vi "Run main.vi"() -> ()   [LabVIEW 2016]
uses:
  Program Files (x86)/National Instruments/LabVIEW 2016/examples/robotics/EPOS2 CANOpen Driver/Low Level VIs/Typedefs/CAN Refnum.ctl
  Program Files (x86)/National Instruments/LabVIEW 2016/examples/robotics/EPOS2 CANOpen Driver/Low Level VIs/Typedefs/CAN Session Pointer.ctl
  Program Files (x86)/National Instruments/LabVIEW 2016/examples/robotics/EPOS2 CANOpen Driver/Low Level VIs/Typedefs/CAN Communication References.ctl
  Program Files (x86)/National Instruments/LabVIEW 2016/examples/robotics/EPOS2 CANOpen Driver/Low Level VIs/Typedefs/kill process notifier array.ctl
  Program Files (x86)/National Instruments/LabVIEW 2016/examples/robotics/EPOS2 CANOpen Driver/Low Level VIs/Typedefs/Write Queue.ctl
  Program Files (x86)/National Instruments/LabVIEW 2016/examples/robotics/EPOS2 CANOpen Driver/Low Level VIs/Typedefs/FPGA CAN Frame Cluster.ctl
  RT/BMS Voltage status 2.ctl
  Tests/BMS Status.ctl
  RT/Pedals Status.ctl
  RT/Clustered SDO.ctl
  RT/Statusword.ctl
  Tests/Dashboard Control.ctl
  RT/Battery Status.ctl
  Tests/Log File Cluster.ctl
  <vilib>/Platform/TimedLoop/XDataNode/timing_clust.ctl
  <vilib>/Platform/TimedLoop/XDataNode/nitl_modes.ctl
  <vilib>/Platform/TimedLoop/XDataNode/wakeup.ctl
  <vilib>/Platform/TimedLoop/XDataNode/XDataNode.xnode
  <vilib>/Platform/TimedLoop/XDataNode/XDNodeRunTimeDep.lvlib
  <vilib>/NI_Real-Time Target Support.lvlib
panel:
  out "Error Notifier":refnum<notifier>
  out "LED Period":i64
  out "LED Color":i16
  out "Last Pedals Update":u32
  in  "Tab Control":T1(tab)
  in  "Don't irritate me":bool=TRUE
  in  "Simulate BMS LV":bool=TRUE
  in  "Simulate Dashboard":bool=TRUE
  in  "Simulate Pedals":bool=TRUE
  in  "Simulate Motors":bool=TRUE
  in  "Simulation Interval":u32=20
  in  "Simulate BMS":bool=TRUE
  in  "\"Pedals\" Status":T2 {"Acceleration pedal" scale=0.0..100.0 scale format="%#_6f%%"; "Break pedal" scale=0.0..100.0 scale format="%#_6f%%"}
  out "Left Motor Status":T3
  out "Target Torque Left":i16(knob) scale=-1000.0..1000.0
  out "Left Motor Statusword":T4
  out "Right Motor Status":T3
  out "Right Motor Statusword":T4
  out "Target Torque Right":i16(knob) scale=1000.0..-1000.0
  out "BMS Status":T5
  out "Battery Status":T6
  out "BMS Low Voltage Status":T7 {"Temp. 0" scale=0.0..80.0; "Temp. 1" scale=0.0..80.0}
  in  "Ready to drive":bool
  in  "Simulate Pumps":bool
  in  "Pumps power":dbl(slide) scale=0.0..100.0 scale format="%#_g%%"
  in  "Dashboard Control":T8={"Tractive System"=TRUE, "RTD"=TRUE, "AMS error"=TRUE, "IMD error"=TRUE, "Low Voltage"=0.0, "High Voltage"=0.0} {"High Voltage" scale=0.0..10.0; "Low Voltage" scale=0.0..10.0}
  in  "Error Listbox":i32(listbox)
  out "Update motors notifier":i32
  out "Update Motors Notifier":refnum<notifier>
  out "Emergency Turn Off Notifier":refnum<notifier>
  out "Pedals status":i32
  out "Update motors":i32
  out "Pool status":i32
  out "Error Queue":refnum<queue>
  out "Shutdown Notifier":refnum<notifier>
  out "Log File Cluster":T9
  out "CAN Session":T11
  out "CANOpen Session":refnum<k20>
  out "Left motor Clustered SDO":T12
  out "Right motor Clustered SDO":T12
  out "State Ring":u16(ring) items=["Init VI", "Init Event Handlers", "Booting sequence", "Operational", "Emergency shutting down", "Shuting down", "Closing VI"]
  in  "Emergency Shutdown Button":bool
  in  "Shutdown Button":bool
  in  "Stop":bool
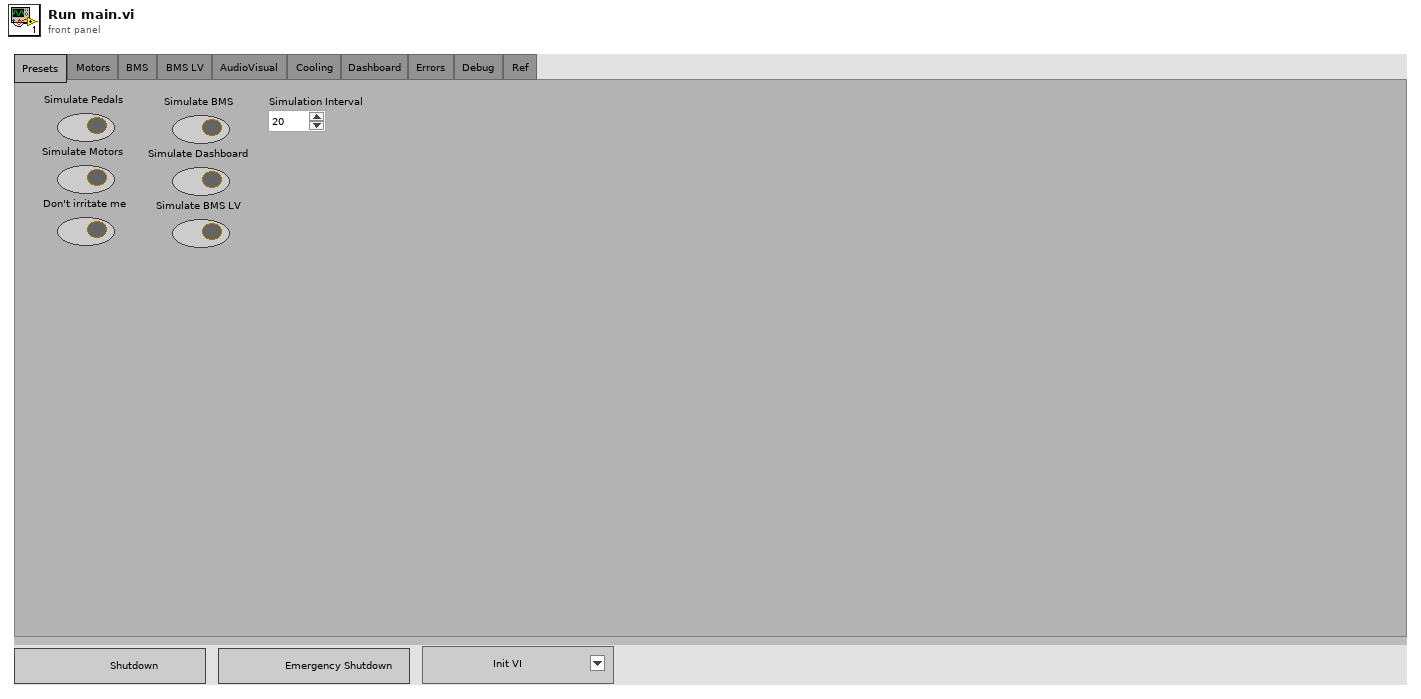
[diagram p1: front panel]
types:
  T1 = enum32{"Presets ", "Motors ", "BMS ", "BMS LV ", "AudioVisual ", "Cooling ", "Dashboard", "Errors ", "Debug ", "Ref "}
  T2 = typedef "Pedals Status.ctl" = cluster{"Acceleration pedal":dbl, "Break pedal":dbl, "Sterring wheel":dbl[unit]}
  T3 = cluster{"Statusword":u16, "Warnings":u16, "Error code":u16, "Error register":u8, "Controller temperature":u8, "Motor temperature":u8, "Troque actual value":i16, "Velocity actual value":i32, "Electric power":u32, "DC current":u32, "Phase A current":u16, "Phase B current":u16, "Electrical Angle":u16}
  T4 = typedef "Statusword.ctl" = cluster{"Ready to switch on":bool, "Switched on":bool, "Operation enabled":bool, "Fault":bool, "Voltage enabled":bool, "Quick stop":bool, "Switch on disabled":bool, "Warning":bool, "Remote":bool, "Target reached":bool, "Internal limit active":bool, "Operation mode specific":bool, "Manufacturer specific":bool}
  T5 = typedef "BMS Status.ctl" = cluster{"INIT":bool, "READY":bool, "WAIT_FOR_ACTIVE":bool, "ACTIVE":bool, "ERROR":bool}
  T6 = typedef "Battery Status.ctl" = cluster{"Hall sensor":i32, "Percent of charge":i16}
  T7 = typedef "BMS Voltage status 2.ctl" = cluster{"Cells Voltage":dbl[], "Temp. 1":u8, "Temp. 0":u8}
  T8 = typedef "Dashboard Control.ctl" = cluster{"Tractive System":bool, "RTD":bool, "AMS error":bool, "IMD error":bool, "Low Voltage":dbl, "High Voltage":dbl}
  T9 = typedef "Log File Cluster.ctl" = cluster{"Log file":refnum<k34>, "semaphore":T10}
  T10 = typedef "Semaphore RefNum" = refnum<k1>
  T11 = typedef "CAN Refnum.ctl" = refnum<k1>
  T12 = typedef "Clustered SDO.ctl" = cluster{"SDO object out":refnum<k20>, "semaphore":T10}
  T13 = typedef "XDNodeRunTimeDep.lvlib/timing_clust.ctl" = cluster{"Expected End [f-1]":u64, "Actual End [f-1]":u64, "Finished Late? [f-1]":bool, "Expected End [i-1]":u64, "Actual End [i-1]":u64, "Finished Late? [i-1]":bool, "Expected Start [i]":u64, "Actual Start [i]":u64, "Expected Start [f]":u64, "Actual Start [f]":u64, "Source Name":string, "Structure Name":string, "Period":i64, "Deadline":i64, "Offset":i64, "Start":i64, "Priority":i32, "Timeout":i32, "Mode":T14, "Wakeup Reason":T15, "Error":errorcluster, "Source Type":string, "Secondary Source Type":string, "Global End Time":u64, "Global Start Time":u64, "Frame Duration":u64, "Iteration Duration":u64, "Assigned CPU":i32, "I/O Scan Engine Mode":u32}
  T14 = typedef "XDNodeRunTimeDep.lvlib/nitl_modes.ctl" = enum32{"No Change", "Process missed periods, maintain original phase", "Discard missed periods, maintain original phase", "Process missed periods, ignore original phase", "Discard missed periods, ignore original phase"}
  T15 = typedef "XDNodeRunTimeDep.lvlib/wakeup.ctl" = enum32{"Normal", "Aborted", "Asynchronous wakeup", "Timing source error", "Timed loop error", "Timeout"}
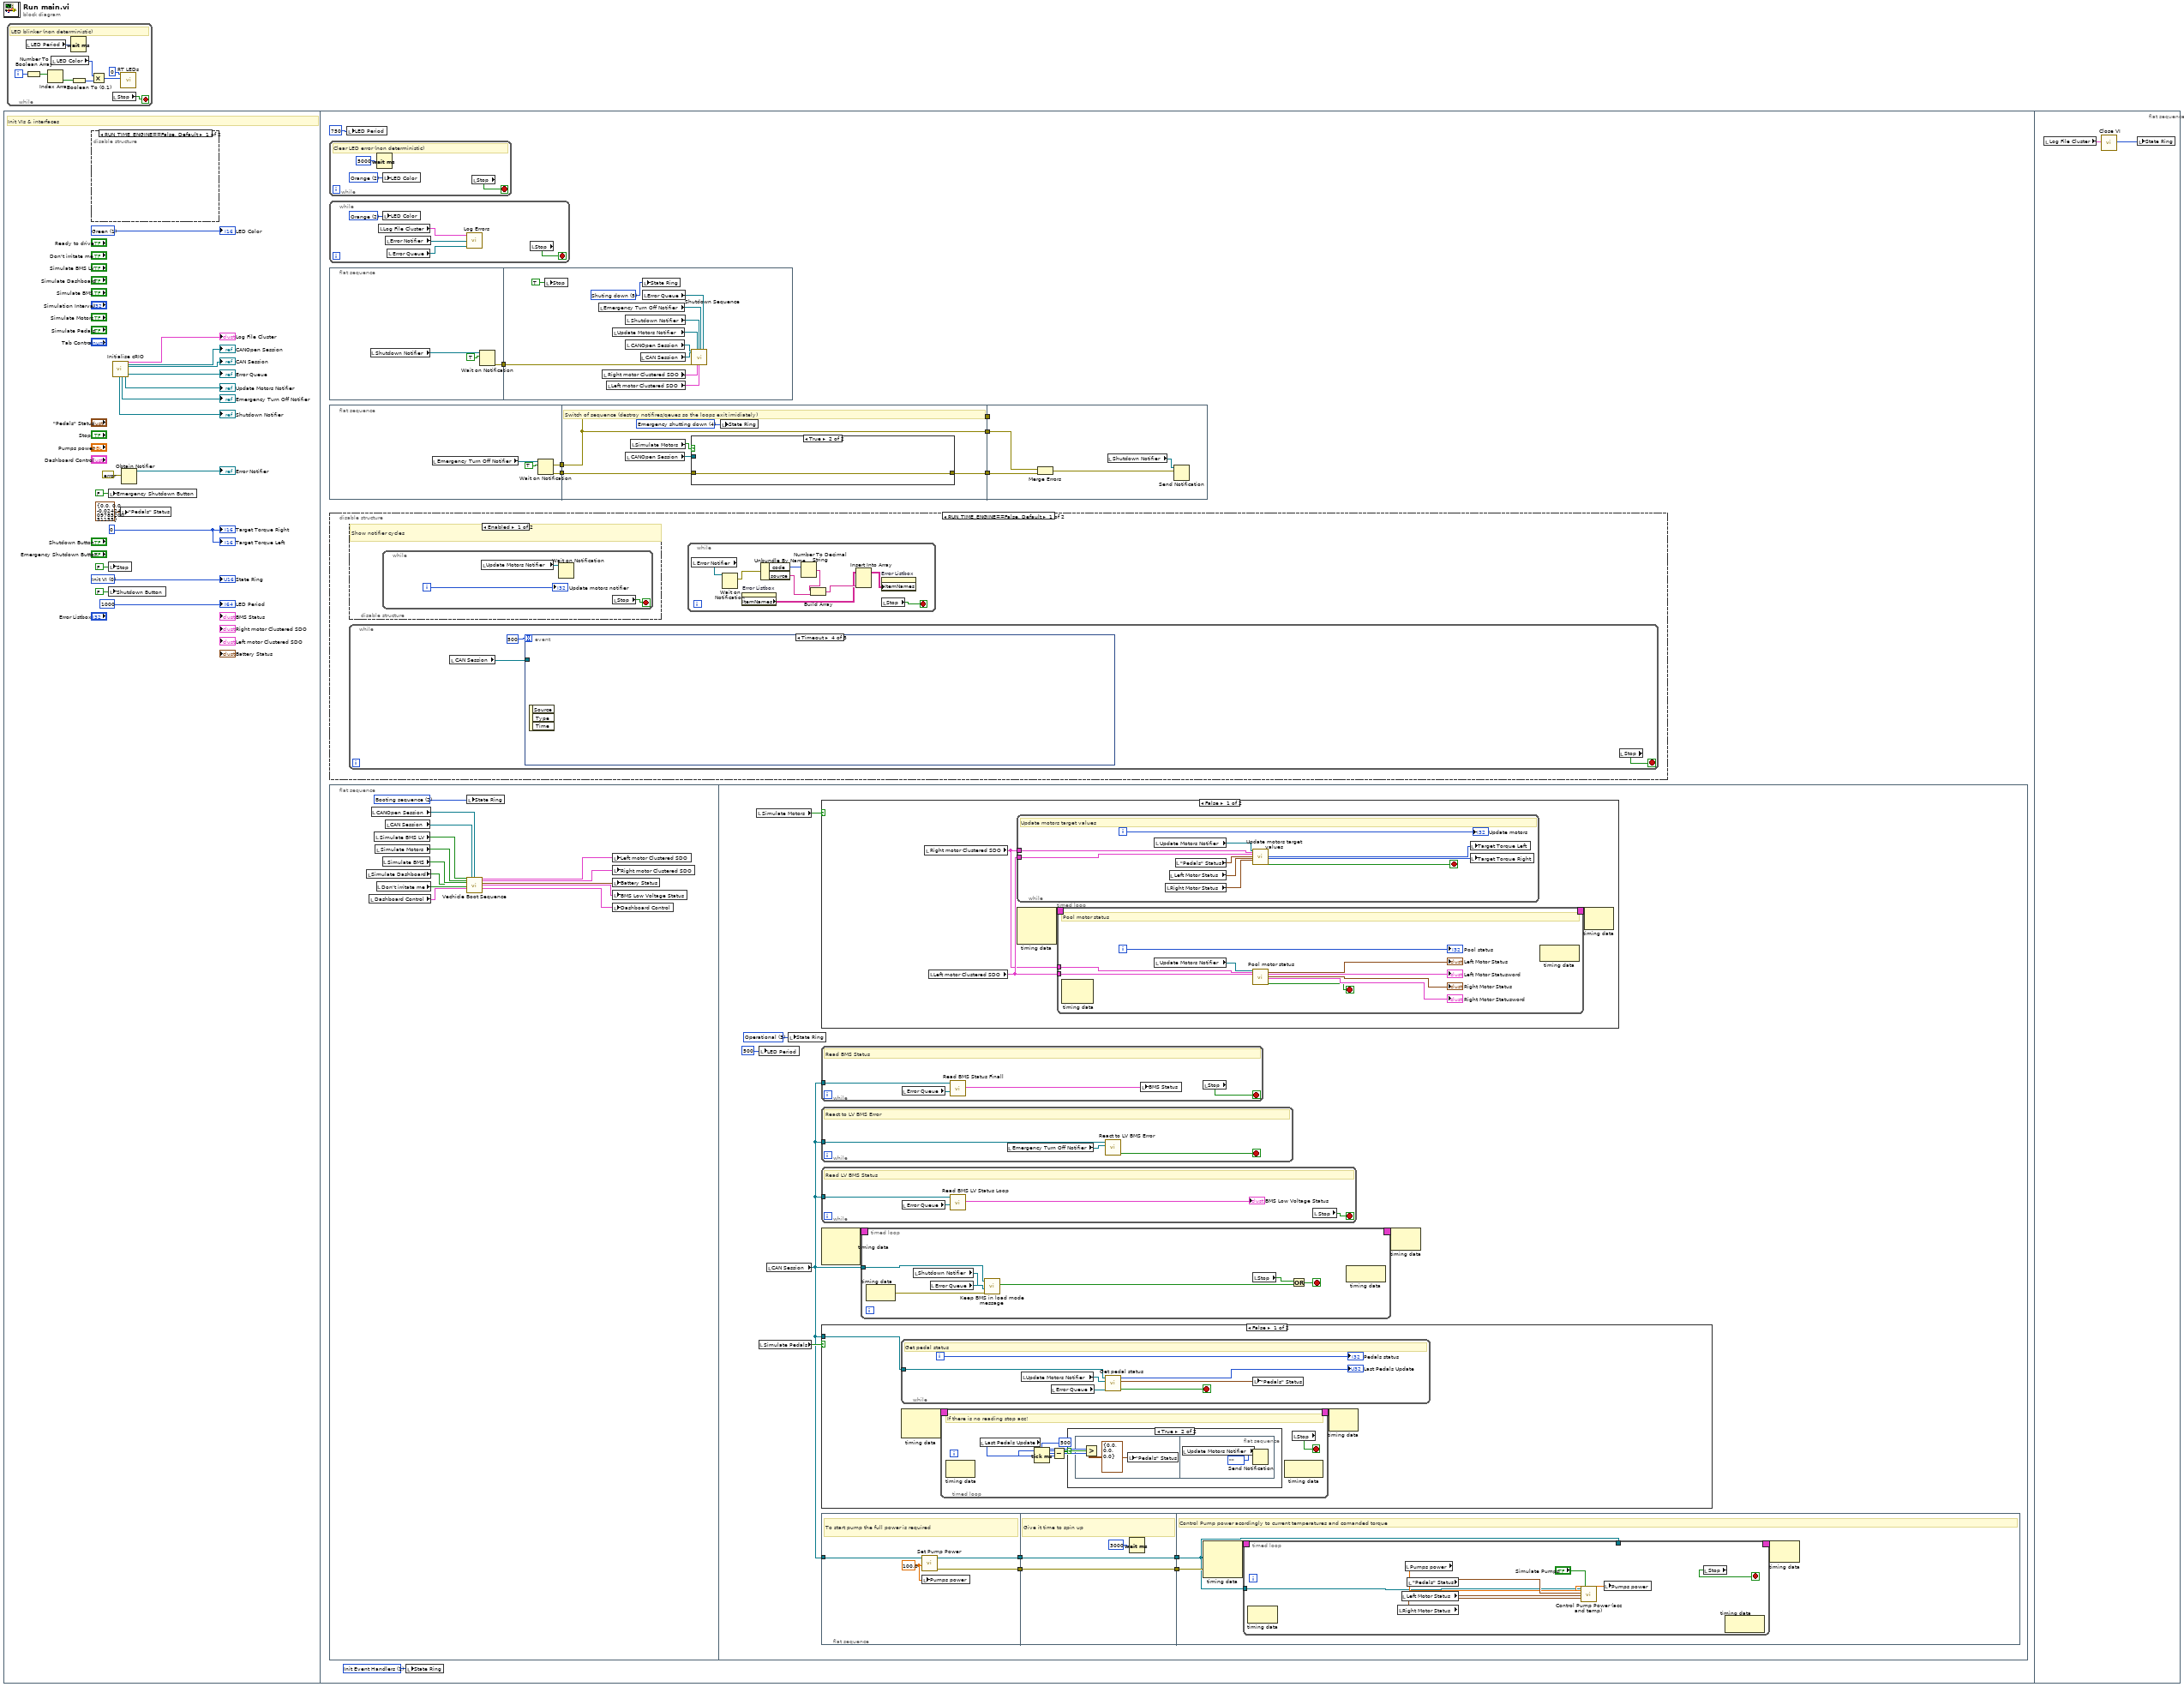
[diagram p0: block diagram]
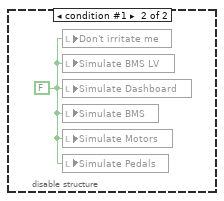
[diagram p2: hidden frame]
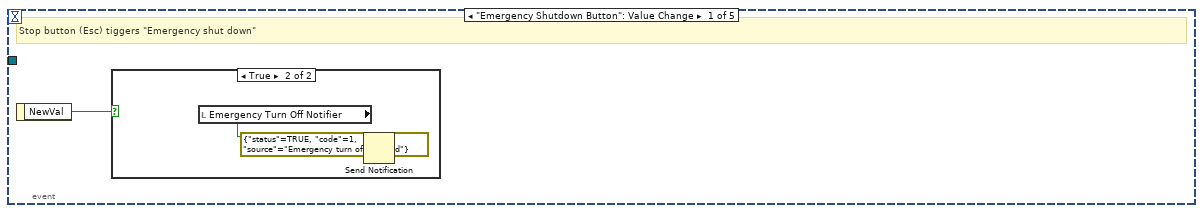
[diagram p4: hidden frame]
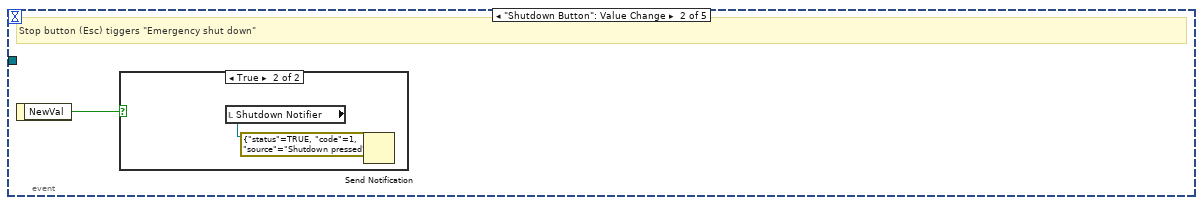
[diagram p6: hidden frame]
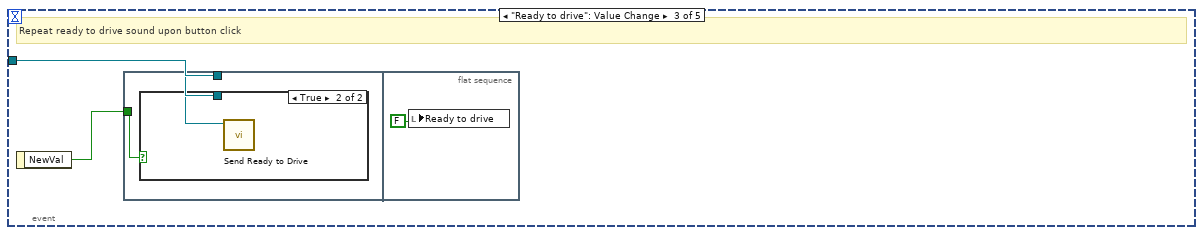
[diagram p8: hidden frame]
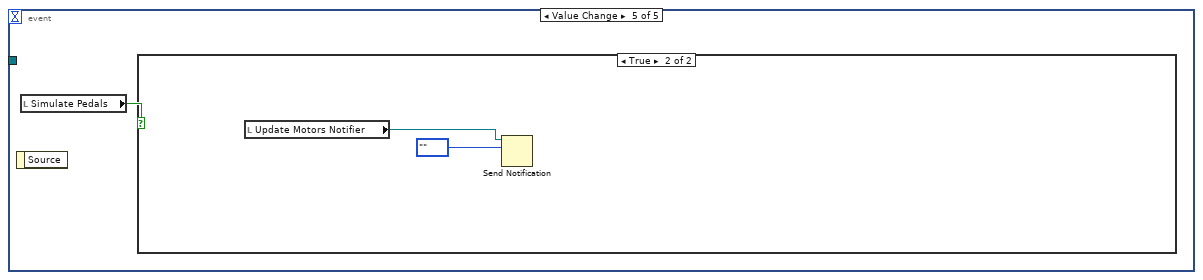
[diagram p10: hidden frame]
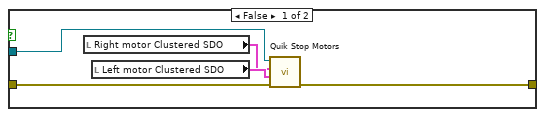
[diagram p13: hidden frame]
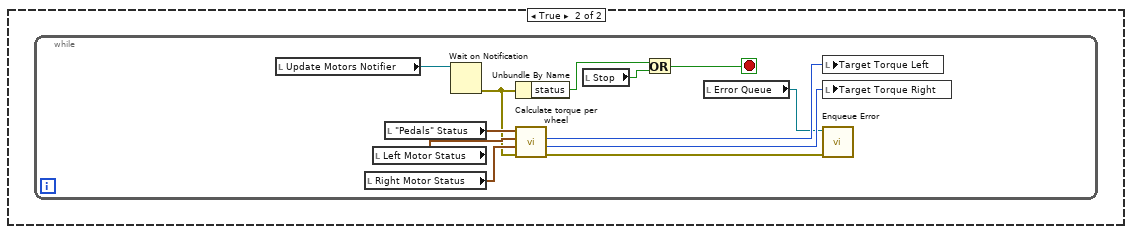
[diagram p16: hidden frame]
diagram:
  n1 = flat-sequence {
    frame #0 {
      w7 = u16 0 items=["Init VI", "Init Event Handlers", "Booting sequence", "Operational", "Emergency shutting down", "Shuting down", "Closing VI"] ("State Ring")
      w9 = u16 1 items=["Green"=1, "Orange"=2]
      w11 = i16 0 ("Target Torque")
      # "Init VIs & interfaces"
      n2 = disable-structure shown="RUN_TIME_ENGINE==False, Default" {
        frame condition #0 (active) {
        }
        frame condition #1 {
          w18 = FALSE ("Don't irritate me")
          n3 = local write "Don't irritate me"(w18) -> ()
          n4 = local write "Simulate BMS LV"(w18) -> ()
          n5 = local write "Simulate Dashboard"(w18) -> ()
          n6 = local write "Simulate BMS"(w18) -> ()
          n7 = local write "Simulate Motors"(w18) -> ()
          n8 = local write "Simulate Pedals"(w18) -> ()
        }
      }
      n9 = local write "Emergency Shutdown Button"(FALSE ("Emergency Shutdown Button")) -> ()
      n10 = local write "Stop"(FALSE ("Stop")) -> ()
      n11 = local write "Shutdown Button"(FALSE ("Shutdown Button")) -> ()
      n12 = call "Initialise cRIO.vi"() -> ("Shutdown Notifier"=→"Shutdown Notifier":refnum<notifier>, "Emergency Turn Off Notifier"=→"Emergency Turn Off Notifier":refnum<notifier>, "Update Motors Notifier"=→"Update Motors Notifier":refnum<notifier>, "Log File Cluster"=→"Log File Cluster":T9, "CANOpen Session"=→"CANOpen Session":refnum<k20>, "CAN Session"=→"CAN Session":T11, "Error Queue"=→"Error Queue":refnum<queue>)  [unwired: 20 in, 1 out]
      n13 = local write "\"Pedals\" Status"(T2 {"Acceleration pedal"=0.0, "Break pedal"=0.0, "Sterring wheel"=-0.024240978520051155} ("\"Pedals\" Status")) -> ()
      n14 = Obtain Notifier(notification data type=errorcluster {"status"=FALSE, "code"=0, "source"=""} ("error constant")) -> (notifier out=→"Error Notifier":refnum<notifier>)  [unwired: 3 in, 2 out]
      "Target Torque Left" <- w11
      "Target Torque Right" <- w11
      "LED Color" <- w9
      "LED Period" <- i64 1000 ("LED Period")
      "State Ring" <- w7
    }
    frame #1 {
      w19 = u16 1 items=["Init VI", "Init Event Handlers", "Booting sequence", "Operational", "Emergency shutting down", "Shuting down", "Closing VI"] ("State Ring")
      n15 = while {
        stop <- w28 stop-if-true
        w29 = u16 2 items=["Green"=1, "Orange"=2]
        # "Clear LED error (non deterministic)"
        n16 = Wait (ms)(milliseconds to wait=u32 5000) -> ()  [unwired: 1 out]
        n17 = local write "LED Color"(w29) -> ()
        n18 = local read "Stop"() -> (w28:bool)
      }
      n19 = while {
        stop <- w34 stop-if-true
        w32 = u16 2 items=["Green"=1, "Orange"=2]
        n20 = local read "Log File Cluster"() -> (w31:T9)
        n21 = local write "LED Color"(w32) -> ()
        n22 = local read "Error Notifier"() -> (w30:refnum<notifier>)
        n23 = local read "Error Queue"() -> (w33:refnum<queue>)
        n24 = call "Log Errors.vi"("Error Queue"=w33, "Error Notifier"=w30, "Log File Cluster"=w31) -> ()  [unwired: 1 in]
        n25 = local read "Stop"() -> (w34:bool)
      }
      n26 = flat-sequence {
        tunnel: [w65] -> w23
        tunnel: w23 -> [w72]
        frame #0 {
          n27 = local read "Shutdown Notifier"() -> (w66:refnum<notifier>)
          n28 = Wait on Notification(notifier=w66, ignore previous (F)=TRUE) -> (error out=w65:errorcluster)  [unwired: 2 in, 3 out]
        }
        frame #1 {
          w68 = u16 5 items=["Init VI", "Init Event Handlers", "Booting sequence", "Operational", "Emergency shutting down", "Shuting down", "Closing VI"] ("State Ring")
          n29 = local write "Stop"(TRUE ("Stop")) -> ()
          n30 = local read "Emergency Turn Off Notifier"() -> (w69:refnum<notifier>)
          n31 = local read "Right motor Clustered SDO"() -> (w73:T12)
          n32 = local read "Left motor Clustered SDO"() -> (w74:T12)
          n33 = local read "Update Motors Notifier"() -> (w76:refnum<notifier>)
          n34 = local read "Shutdown Notifier"() -> (w75:refnum<notifier>)
          n35 = local read "CANOpen Session"() -> (w78:refnum<k20>)
          n36 = local read "CAN Session"() -> (w77:T11)
          n37 = local write "State Ring"(w68) -> ()
          n38 = local read "Error Queue"() -> (w71:refnum<queue>)
          n39 = call "Shutdown Sequence.vi"("CANOpen Session"=w78, "CAN Session"=w77, "error in (no error)"=w72, "Update Motors Notifier"=w76, "Right motor Clustered SDO"=w73, "Shutdown Notifier"=w75, "Left motor Clustered SDO"=w74, "Emergency Turn Off Notifier"=w69, "Error Queue"=w71) -> ()  [unwired: 18 in, 1 out]
        }
      }
      n40 = flat-sequence {
        tunnel: [w81] -> w26
        tunnel: [w80] -> w25
        tunnel: w26 -> [w86]
        tunnel: w25 -> [w84]
        tunnel: [w84] -> w24
        tunnel: [w85] -> w22
        tunnel: [w84] -> w21
        tunnel: w24 -> [_]
        tunnel: w22 -> [w97]
        tunnel: w21 -> [w96]
        frame #0 {
          n41 = local read "Emergency Turn Off Notifier"() -> (w82:refnum<notifier>)
          n42 = Wait on Notification(notifier=w82, ignore previous (F)=TRUE) -> (notification=w80:errorcluster, error out=w81:errorcluster)  [unwired: 2 in, 2 out]
        }
        frame #1 {
          w83 = u16 4 items=["Init VI", "Init Event Handlers", "Booting sequence", "Operational", "Emergency shutting down", "Shuting down", "Closing VI"] ("State Ring")
          # "Switch of sequence (destroy notifires/qeues so the loops exit imidiately)"
          n43 = local read "CANOpen Session"() -> (w87:refnum<k20>)
          n44 = local read "Simulate Motors"() -> (w88:bool)
          n45 = case shown="True" w88 {
            tunnel: w87 -> [w93 _]
            tunnel: w86 -> [w92 w94]
            tunnel: [w89 w94] -> w85
            frame False {
              n46 = local read "Right motor Clustered SDO"() -> (w90:T12)
              n47 = local read "Left motor Clustered SDO"() -> (w91:T12)
              n48 = call "Quik Stop Motors.vi"("error in (no error)"=w92, "Left motor Clustered SDO"=w91, "Right motor Clustered SDO"=w90, "CANOpen session"=w93) -> ("error out"=w89:errorcluster)  [unwired: 5 in, 2 out]
            }
            frame True {
            }
          }
          n49 = local write "State Ring"(w83) -> ()
        }
        frame #2 {
          n50 = Merge Errors(w96, w97) -> (w95:errorcluster)
          n51 = local read "Shutdown Notifier"() -> (w98:refnum<notifier>)
          n52 = Send Notification(notification=w95, notifier=w98) -> ()  [unwired: 1 in, 2 out]
        }
      }
      n53 = disable-structure shown="RUN_TIME_ENGINE==False, Default" {
        frame condition #0 (active) {
          n54 = disable-structure shown="Enabled" {
            frame Enabled {
              # "Show notifier cycles"
              n55 = while {
                i -> [w44]
                stop <- w45 stop-if-true
                n56 = local read "Update Motors Notifier"() -> (w46:refnum<notifier>)
                n57 = Wait on Notification(notifier=w46) -> ()  [unwired: 3 in, 4 out]
                n58 = local read "Stop"() -> (w45:bool)
                "Update motors notifier" <- w44
              }
            }
            frame Disabled {
            }
          }
          n59 = while {
            stop <- w48 stop-if-true
            n60 = local read "CAN Session"() -> (w49:T11)
            n61 = event shown="[3] Timeout" {
              selector: _ -> [_ _ _ _ _]
              dyn-events: _ -> [_ _ _ _ _]
              timeout: 500 -> [_ _ _ _ _]
              tunnel: w49 -> [_ _ w56 _ _]
              event "Emergency Shutdown Button": Value Change {
                # "Stop button (Esc) tiggers \"Emergency shut down\""
                n62 = event-data() -> ("NewVal"=w50:bool)  [unwired: 1 in]
                n63 = case shown="True" w50 {
                  frame False {
                  }
                  frame True {
                    n64 = local read "Emergency Turn Off Notifier"() -> (w52:refnum<notifier>)
                    n65 = Send Notification(notification=errorcluster {"status"=TRUE, "code"=1, "source"="Emergency turn off pressed"}, notifier=w52) -> ()  [unwired: 1 in, 2 out]
                  }
                }
              }
              event "Shutdown Button": Value Change {
                # "Stop button (Esc) tiggers \"Emergency shut down\""
                n66 = event-data() -> ("NewVal"=w53:bool)  [unwired: 1 in]
                n67 = case shown="True" w53 {
                  frame False {
                  }
                  frame True {
                    n68 = local read "Shutdown Notifier"() -> (w55:refnum<notifier>)
                    n69 = Send Notification(notification=errorcluster {"status"=TRUE, "code"=1, "source"="Shutdown pressed"}, notifier=w55) -> ()  [unwired: 1 in, 2 out]
                  }
                }
              }
              event "Ready to drive": Value Change {
                # "Repeat ready to drive sound upon button click"
                n70 = event-data() -> ("NewVal"=w57:bool)  [unwired: 1 in]
                n71 = flat-sequence {
                  tunnel: w57 -> [w59]
                  tunnel: w56 -> [w58]
                  frame #0 {
                    n72 = case shown="True" w59 {
                      tunnel: w58 -> [_ w60]
                      frame False {
                      }
                      frame True {
                        n73 = call "Send Ready to Drive.vi"("CAN Session In"=w60) -> ()  [unwired: 9 in, 2 out]
                      }
                    }
                  }
                  frame #1 {
                    n74 = local write "Ready to drive"(FALSE ("Ready to drive")) -> ()
                  }
                }
              }
              event Timeout {
                n75 = event-data() -> ()  [unwired: 1 in, 3 out]
              }
              event Value Change {
                n76 = event-data() -> ()  [unwired: 1 in, 1 out]
                n77 = local read "Simulate Pedals"() -> (w62:bool)
                n78 = case shown="True" w62 {
                  frame False {
                  }
                  frame True {
                    n79 = local read "Update Motors Notifier"() -> (w63:refnum<notifier>)
                    n80 = Send Notification(notification=enum16{""}."", notifier=w63) -> ()  [unwired: 1 in, 2 out]
                  }
                }
              }
            }
            n81 = local read "Stop"() -> (w48:bool)
          }
          n82 = while {
            stop <- w35 stop-if-true
            n83 = local read "Error Notifier"() -> (w43:refnum<notifier>)
            n84 = Wait on Notification(notifier=w43) -> (notification=w42:errorcluster)  [unwired: 3 in, 3 out]
            n85 = property on="Error Listbox" class="MCListbox (strict)"() -> ("ItemNames"=w37:string[][])  [unwired: 2 in, 2 out]
            n86 = Unbundle By Name(w42) -> ("code"=w39:i32, "source"=w41:string)
            n87 = Number To Decimal String(number=w39) -> (decimal integer string=w40:string)  [unwired: 1 in]
            n88 = Build Array(w40, w41) -> (w38:string[])
            n89 = Insert Into Array(array=w37, new element=w38) -> (w36:string[][])  [unwired: 2 in]
            n90 = property on="Error Listbox" class="MCListbox (strict)"("ItemNames"=w36) -> ()  [unwired: 2 in, 2 out]
            n91 = local read "Stop"() -> (w35:bool)
          }
        }
        frame condition #1 {
        }
      }
      n92 = flat-sequence {
        frame #0 {
          w99 = u16 2 items=["Init VI", "Init Event Handlers", "Booting sequence", "Operational", "Emergency shutting down", "Shuting down", "Closing VI"] ("State Ring")
          n93 = local read "Simulate Dashboard"() -> (w109:bool)
          n94 = local read "Dashboard Control"() -> (w101:T8)
          n95 = local read "CANOpen Session"() -> (w106:refnum<k20>)
          n96 = local read "Simulate BMS LV"() -> (w112:bool)
          n97 = local read "Simulate Motors"() -> (w110:bool)
          n98 = local read "Don't irritate me"() -> (w108:bool)
          n99 = local read "Simulate BMS"() -> (w111:bool)
          n100 = local read "CAN Session"() -> (w107:T11)
          n101 = local write "State Ring"(w99) -> ()
          n102 = call "Vechicle Boot Sequence.vi"("Simulate BMS LV"=w112, "Simulate Motors"=w110, "Simulate BMS"=w111, "Simulate Dashboard"=w109, "Don't irritate me"=w108, "Dashboard Control in"=w101, "CAN Session"=w107, "CANOpen Session"=w106) -> ("Left motor Clustered SDO"=w104:T12, "Right motor Clustered SDO"=w105:T12, "Battery Status"=w103:T6, "BMS Low Voltage Status"=w100:T7, "Dashboard Control out"=w102:T8)  [unwired: 14 in, 1 out]
          n103 = local write "Left motor Clustered SDO"(w104) -> ()
          n104 = local write "Right motor Clustered SDO"(w105) -> ()
          n105 = local write "Battery Status"(w103) -> ()
          n106 = local write "BMS Low Voltage Status"(w100) -> ()
          n107 = local write "Dashboard Control"(w102) -> ()
        }
        frame #1 {
          w113 = u16 3 items=["Init VI", "Init Event Handlers", "Booting sequence", "Operational", "Emergency shutting down", "Shuting down", "Closing VI"] ("State Ring")
          n108 = local read "Simulate Motors"() -> (w117:bool)
          n109 = local read "Simulate Pedals"() -> (w116:bool)
          n110 = local write "LED Period"(i64 500 ("LED Period")) -> ()
          n111 = local read "CAN Session"() -> (w115:T11)
          n112 = local write "State Ring"(w113) -> ()
          n113 = case shown="False" w117 {
            frame False {
              n114 = local read "Right motor Clustered SDO"() -> (w195:T12)
              n115 = local read "Left motor Clustered SDO"() -> (w196:T12)
              n116 = while {
                tunnel: w196 -> [w218]
                tunnel: w195 -> [w219]
                i -> [w221]
                stop <- w212 stop-if-true
                # "Update motors target values"
                n117 = local read "Update Motors Notifier"() -> (w220:refnum<notifier>)
                n118 = local read "Right Motor Status"() -> (w215:T3)
                n119 = local read "Left Motor Status"() -> (w216:T3)
                n120 = local read "\"Pedals\" Status"() -> (w217:T2)
                n121 = call "Update motors target values.vi"("Update Motors Notifier"=w220, "Right motor Clustered SDO"=w219, "Left motor Clustered SDO"=w218, "\"Pedals\" Status"=w217, "Left Motor Status"=w216, "Right Motor Status"=w215) -> ("Target Torque Left"=w214:i16, "Target Torque Right"=w213:i16, "Exit?"=w212:bool)  [unwired: 19 in]
                n122 = local write "Target Torque Left"(w214) -> ()
                n123 = local write "Target Torque Right"(w213) -> ()
                "Update motors" <- w221
              }
              n124 = node-c288() -> (w198:T13)  [unwired: 3 in]
              n125 = timed-loop {
                timing: w198 -> [_]
                timing-out: [_] -> w197
                tunnel: w196 -> [w206]
                tunnel: w195 -> [w205]
                i -> [w207]
                stop <- w199 stop-if-true
                # "Pool motor status"
                n126 = node-c288() -> ()  [unwired: 1 in, 2 out]
                n127 = local read "Update Motors Notifier"() -> (w204:refnum<notifier>)
                n128 = call "Pool motor status.vi"("Update Motors Notifier"=w204, "Right motor Clustered SDO"=w205, "Left motor Clustered SDO"=w206) -> ("Left Motor Status"=→"Left Motor Status":T3, "Left Motor Statusword"=→"Left Motor Statusword":T4, "Right Motor Status"=→"Right Motor Status":T3, "Right Motor Statusword"=→"Right Motor Statusword":T4, "Exit?"=w199:bool)  [unwired: 20 in]
                n129 = node-c288() -> ()  [unwired: 1 in, 1 out]
                "Pool status" <- w207
              }
              n130 = node-c288(w197) -> ()  [unwired: 1 out]
            }
            frame True {
              n131 = while {
                stop <- w229 stop-if-true
                n132 = local read "Update Motors Notifier"() -> (w231:refnum<notifier>)
                n133 = local read "Right Motor Status"() -> (w226:T3)
                n134 = local read "Left Motor Status"() -> (w227:T3)
                n135 = local read "\"Pedals\" Status"() -> (w228:T2)
                n136 = Wait on Notification(notifier=w231) -> (error out=w222:errorcluster)  [unwired: 3 in, 3 out]
                n137 = Unbundle By Name(w222) -> ("status"=w223:bool)
                n138 = call "Calculate torque per wheel.vi"("Error In"=w222, "Right Motor Status"=w226, "Left Motor Status"=w227, "\"Pedals\" Status"=w228) -> ("Error Out"=w225:errorcluster, "Target Torque Right"=w232:i16, "Target Torque Left"=w233:i16)  [unwired: 5 in]
                n139 = local read "Stop"() -> (w230:bool)
                n140 = Or(x=w223, y=w230) -> (x .or. y?=w229:bool)
                n141 = local read "Error Queue"() -> (w224:refnum<queue>)
                n142 = local write "Target Torque Left"(w233) -> ()
                n143 = local write "Target Torque Right"(w232) -> ()
                n144 = call "Enqueue Error.vi"("error in"=w225, "Error Queue"=w224) -> ()  [unwired: 10 in]
              }
            }
          }
          n145 = while {
            tunnel: w115 -> [w126]
            stop <- w125 stop-if-true
            # "Read BMS Status"
            n146 = local read "Error Queue"() -> (w124:refnum<queue>)
            n147 = call "Read BMS Status Finall.vi"("Error Queue"=w124, "CAN Session In"=w126) -> ("BMS Status"=w127:T5)  [unwired: 8 in, 1 out]
            n148 = local write "BMS Status"(w127) -> ()
            n149 = local read "Stop"() -> (w125:bool)
          }
          n150 = while {
            tunnel: w115 -> [w180]
            stop <- w182 stop-if-true
            # "React to LV BMS Error"
            n151 = local read "Emergency Turn Off Notifier"() -> (w181:refnum<notifier>)
            n152 = call "React to LV BMS Error.vi"("Emergency Turn Off Notifier"=w181, "CAN Session In"=w180) -> ("Exit?"=w182:bool)  [unwired: 8 in, 1 out]
          }
          n153 = while {
            tunnel: w115 -> [w130]
            stop <- w128 stop-if-true
            # "Read LV BMS Status"
            n154 = local read "Error Queue"() -> (w129:refnum<queue>)
            n155 = call "Read BMS LV Status Loop.vi"("Error Queue"=w129, "CAN Session In"=w130) -> ("BMS Low Voltage Status"=→"BMS Low Voltage Status":T7)  [unwired: 8 in, 1 out]
            n156 = local read "Stop"() -> (w128:bool)
          }
          n157 = node-c288() -> (w123:T13)  [unwired: 3 in]
          n158 = case shown="False" w116 {
            tunnel: w115 -> [w157 _]
            frame False {
              n159 = while {
                tunnel: w157 -> [w173]
                i -> [w179]
                stop <- w174 stop-if-true
                # "Get pedal status"
                n160 = local read "Update Motors Notifier"() -> (w176:refnum<notifier>)
                n161 = local read "Error Queue"() -> (w177:refnum<queue>)
                n162 = call "Get pedal status.vi"("Error Queue"=w177, "Update Motors Notifier"=w176, "CAN Session In"=w173) -> ("Exit?"=w174:bool, "\"Pedals\" Status"=w175:T2, "Last Pedals Update"=→"Last Pedals Update":u32)  [unwired: 6 in]
                n163 = local write "\"Pedals\" Status"(w175) -> ()
                "Pedals status" <- w179
              }
              n164 = node-c288() -> (w159:T13)  [unwired: 2 in]
              n165 = timed-loop {
                timing: w159 -> [_]
                timing-out: [_] -> w158
                stop <- w160 stop-if-true
                # "If there is no reading stop acc!"
                n166 = node-c288() -> ()  [unwired: 1 in, 1 out]
                n167 = local read "Last Pedals Update"() -> (w164:u32)
                n168 = Tick Count (ms)() -> (millisecond timer value=w165:u32)
                n169 = Subtract(x=w165, y=w164) -> (x-y=w163:u32)
                n170 = Greater?(x=w163, y=u32 500) -> (0:w161:bool)
                n171 = case shown="True" w161 {
                  frame False {
                  }
                  frame True {
                    n172 = flat-sequence {
                      frame #0 {
                        n173 = local write "\"Pedals\" Status"(T2 {"Acceleration pedal"=0.0, "Break pedal"=0.0, "Sterring wheel"=0.0} ("\"Pedals\" Status")) -> ()
                      }
                      frame #1 {
                        n174 = local read "Update Motors Notifier"() -> (w167:refnum<notifier>)
                        n175 = Send Notification(notification=enum16{""}."", notifier=w167) -> ()  [unwired: 1 in, 2 out]
                      }
                    }
                  }
                }
                n176 = node-c288() -> ()  [unwired: 1 in, 1 out]
                n177 = local read "Stop"() -> (w160:bool)
              }
              n178 = node-c288(w158) -> ()  [unwired: 1 out]
            }
            frame True {
            }
          }
          n179 = flat-sequence {
            tunnel: [w135] -> w121
            tunnel: [w134] -> w120
            tunnel: w115 -> [w132]
            tunnel: w121 -> [w137]
            tunnel: [w137] -> w119
            tunnel: [w136] -> w118
            tunnel: w120 -> [w136]
            tunnel: w119 -> [w139]
            tunnel: w118 -> [w140]
            frame #0 {
              w133 = 100.0 ("Power %")
              # "To start pump the full power is required"
              n180 = call "Set Pump Power.vi"("Power %"=w133, "CAN Session In"=w132) -> ("error out"=w134:errorcluster, "CAN Session Out"=w135:T11)  [unwired: 8 in]
              n181 = local write "Pumps power"(w133) -> ()
            }
            frame #1 {
              # "Give it time to spin up"
              n182 = Wait (ms)(milliseconds to wait=u32 3000) -> ()  [unwired: 1 out]
            }
            frame #2 {
              # "Control Pump power acordingly to current temperatures and comanded torque"
              n183 = node-c288(w140) -> (w142:T13)  [unwired: 2 in]
              n184 = timed-loop {
                timing: w142 -> [_]
                timing-out: [_] -> w141
                tunnel: w139 -> [_]
                tunnel: w139 -> [w144]
                stop <- w143 stop-if-true
                n185 = node-c288() -> ()  [unwired: 1 in, 1 out]
                n186 = local read "Right Motor Status"() -> (w148:T3)
                n187 = local read "Left Motor Status"() -> (w149:T3)
                n188 = local read "Pumps power"() -> (w146:dbl)
                n189 = local read "\"Pedals\" Status"() -> (w150:T2)
                n190 = call "Control Pump Power (acc and temp).vi"("CAN Session In"=w144, "Pumps power in"=w146, "\"Pedals\" Status"=w150, "Left Motor Status"=w149, "Right Motor Status"=w148, "Simulate Pumps"="Simulate Pumps") -> ("Pumps power out"=w145:dbl)  [unwired: 11 in, 2 out]
                n191 = local write "Pumps power"(w145) -> ()
                n192 = local read "Stop"() -> (w143:bool)
                n193 = node-c288() -> ()  [unwired: 1 in, 1 out]
              }
              n194 = node-c288(w141) -> ()  [unwired: 1 out]
            }
          }
          n195 = timed-loop {
            timing: w123 -> [_]
            timing-out: [_] -> w122
            tunnel: w115 -> [w188]
            stop <- w183 stop-if-true
            n196 = node-c288() -> (w189:errorcluster)  [unwired: 1 in]
            n197 = local read "Shutdown Notifier"() -> (w184:refnum<notifier>)
            n198 = local read "Error Queue"() -> (w185:refnum<queue>)
            n199 = call "Keep BMS in load mode message.vi"("error in"=w189, "Error Queue"=w185, "Shutdown Notifier"=w184, "CAN Session In"=w188) -> ("Exit?"=w187:bool)  [unwired: 6 in, 1 out]
            n200 = local read "Stop"() -> (w186:bool)
            n201 = Or(x=w186, y=w187) -> (x .or. y?=w183:bool)
            n202 = node-c288() -> ()  [unwired: 1 in, 1 out]
          }
          n203 = node-c288(w122) -> ()  [unwired: 1 out]
        }
      }
      n204 = local write "LED Period"(i64 750 ("LED Period")) -> ()
      n205 = local write "State Ring"(w19) -> ()
    }
    frame #2 {
      n206 = local read "Log File Cluster"() -> (w234:T9)
      n207 = call "Close VI.vi"("Log File Cluster"=w234) -> ("State Ring"=w235:u16)  [unwired: 10 in]
      n208 = local write "State Ring"(w235) -> ()
    }
  }
  n209 = while {
    i -> [w242]
    stop <- w244 stop-if-true
    # "LED blinker (non deterministic)"
    n210 = local read "LED Period"() -> (w236:i64)
    n211 = Number To Boolean Array(number=w242) -> (Boolean array=w241:bool[])
    n212 = Index Array(array=w241) -> (element=w240:bool)  [unwired: 1 in]
    n213 = local read "LED Color"() -> (w238:i16)
    n214 = Wait (ms)(milliseconds to wait=w236) -> ()  [unwired: 1 out]
    n215 = Boolean To (0,1)(Boolean=w240) -> (0, 1=w239:i16)
    n216 = Multiply(x=w238, y=w239) -> (x*y=w237:i16)
    n217 = local read "Stop"() -> (w244:bool)
    n218 = call <vilib>:"RT LEDs.vi"("State"=w237, "LED Num"=0) -> ()  [unwired: 4 in, 2 out]
  }
